vi "Read Profile Buf Size(for High Speed Communication).vi"(8 "error in (no error)":errorcluster, 11 "Device ID (0)":i32) -> (0 "error out":errorcluster, 2 "Profile Buf Size":u32, 3 "Device ID out":i32)   [LabVIEW 2010, in "KEYENCE LJ-X8000A.lvlib"]
uses:
  KEYENCE LJ-X8000A.lvlib
panel:
  # "(c) 2012 KEYENCE CORPORATION.  ALL RIGHTS RESERVED."
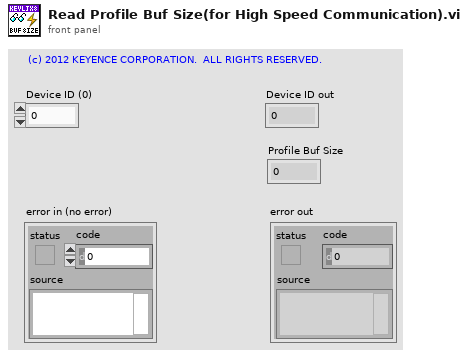
[diagram p1: front panel]
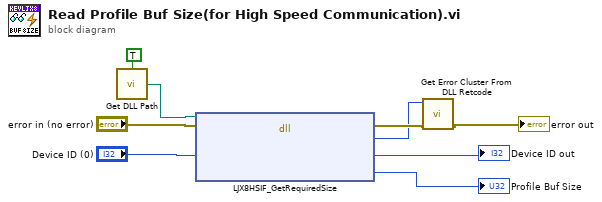
[diagram p0: block diagram]
diagram:
  n1 = call "Get DLL Path.vi"("isWrapperDLL (False)"=TRUE) -> ("DLL Path"=w4:path)  [unwired: 2 in]
  n2 = dll-call lib="C:/bukken/S151/TFS/soft/src/Product/Dev/LVDriver/KEYENCE LJ-X8000/LJX8_HighSpeedWrapper.*" fn="LJX8HSIF_GetRequiredSize"(path in=w4, error in="error in (no error)", "lDeviceId"="Device ID (0)") -> (error out=w3:errorcluster, "lRetCode"=w2:i32, "lDeviceId"=→"Device ID out":i32, "pdwProfileSize"=→"Profile Buf Size":u32)  [unwired: 2 in, 1 out]
  n3 = call "Get Error Cluster From DLL Retcode.vi"("error in (no error)"=w3, "DLL Return Code"=w2) -> ("error out"=→"error out":errorcluster)  [unwired: 8 in, 1 out]
